vi "Unflatten Layers.vi"(8 "Error In":errorcluster, 11 "String":string) -> (0 "Error Out":errorcluster, 3 "Layers":refnum<class "Layer.lvclass">[](array[class]))   [LabVIEW 2021]
uses:
  <vilib>/LabVIEW Icon API/lv_icon/Classes/Layer/Layer.lvclass
  <vilib>/LabVIEW Icon API/lv_icon/lv_icon.lvlib
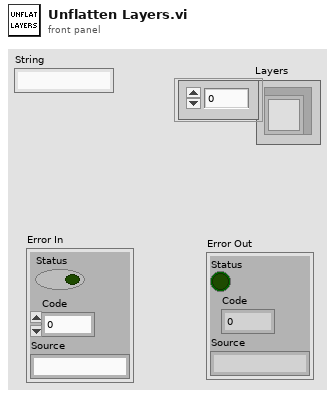
[diagram p1: front panel]
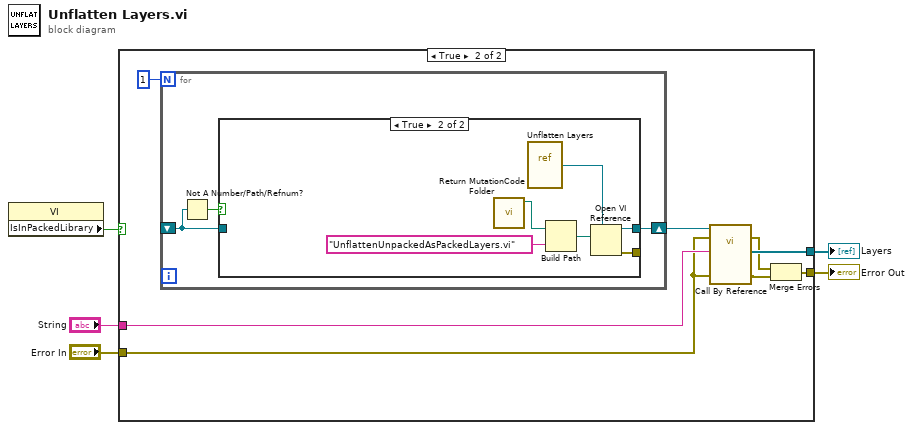
[diagram p0: block diagram]
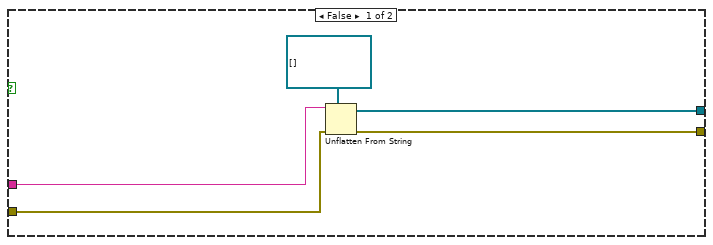
[diagram p2: hidden frame]
diagram:
  n1 = property class="VI"() -> ("IsInPackedLibrary"=w1:bool)  [unwired: 2 in, 2 out]
  n2 = case shown="True" w1 {
    tunnel: "String" -> [w6 w16]
    tunnel: [w8 w15] -> w4
    tunnel: "Error In" -> [w7 w14]
    tunnel: [w9 w11] -> w2
    frame False {
      n3 = Unflatten From String(type=refnum<class "Layer.lvclass">[] [] ("Layers"), binary string=w6, error in (no error)=w7) -> (value=w8:refnum<class "Layer.lvclass">[], error out=w9:errorcluster)  [unwired: 2 in, 1 out]
    }
    frame True {
      n4 = for {
        N: 1 -> [_]
        shift-right: [w19] -> w17
        shift-left: _ -> [w20]
        n5 = Not A Number/Path/Refnum?(number/path/refnum=w20) -> (NaN/Path/Refnum?=w21:bool)
        n6 = case shown="True" w21 {
          tunnel: [w22 w26] -> w19
          tunnel: w20 -> [w22 _]
          tunnel: [_ w24] -> _
          frame False {
          }
          frame True {
            n7 = call <vilib>:"Return MutationCode Folder.vi"() -> ("Base Path Mutation Code"=w25:path)  [unwired: 11 in]
            n8 = vi-ref <resource>:"Unflatten Layers.vi"() -> (w23:refnum<vi>)
            n9 = Build Path(base path=w25, name or relative path="UnflattenUnpackedAsPackedLayers.vi") -> (appended path=w27:path)
            n10 = Open VI Reference(type specifier VI Refnum (for type only)=w23, vi path=w27) -> (vi reference=w26:refnum<vi>, error out=w24:errorcluster)  [unwired: 4 in]
          }
        }
      }
      n11 = call-by-ref "?"(reference=w17, error in=w14, "Error In"=w14, "String"=w16) -> (error out=w13:errorcluster, "Error Out"=w12:errorcluster, "Layers"=w15:refnum<class "Layer.lvclass">[])  [unwired: 8 in, 1 out]
      n12 = Merge Errors(w13, w12) -> (w11:errorcluster)
    }
  }
  "Error Out" <- w2
  "Layers" <- w4
